vi "HighPassFilter.vi"(10 "Data":waveform(dbl)={"t0"=timestamp(3769531068.022168 s since 1904-01-01), "dt"=2.0833333333333333e-05, "Y"=array[14400 elements]}, 11 "Settings":T1={"Name of test"="Colin--Colin 01", "Date"=timestamp(3769531010.377861 s since 1904-01-01), "Location"="Home", "Template"="Acoustic Test", "Soundcard"="485B39 200083408035100798118210422", "resolution"=32, "Sampling rate"=48000, "Ch1 Gain "=0.0, "Ch2 Gain"=0.0, "Sample time (s)"=0.3, "Pre-trigger (s)"=0.001, "Hammer Threshold"=0.3, "Positions"=1, "Taps/Position"=5, "Set Names"="H", "Freq resolution"=1.0, "Hammer cutoff"=1.0, "Mic cutoff"=1.0, "Double bounce "=0.1, "Hammer Cal"=23.6, "dB Offset"=0.0, "Accel Cal"=1.0, "Vibrometer Cal"=40.0, "Mic Cal"=66.0, "Output"=2, "Voltage Cal"=1.0, "Vibrometer Port"="ASRL27::INSTR", "Range"=20, "High Pass"=2, "Bandwidth"=25, "X Range"=[{"Minimum"=200.0, "Maximum"=10000.0, "Increment"=10.0, "Minor Increment"=100.0, "Start"=200.0}, {"Minimum"=0.0005291005, "Maximum"=0.02, "Increment"=0.01, "Minor Increment"=0.001, "Start"=0.01}, {"Minimum"=0.0, "Maximum"=0.3, "Increment"=0.1, "Minor Increment"=0.01, "Start"=0.0}, {"Minimum"=200.0, "Maximum"=10000.0, "Increment"=10.0, "Minor Increment"=100.0, "Start"=1000.0}], "Y Range"=[{"Minimum"=-25.0, "Maximum"=0.0, "Increment"=5.0, "Minor Increment"=1.0, "Start"=-25.0}, {"Minimum"=-0.001, "Maximum"=0.01, "Increment"=0.002, "Minor Increment"=0.0005, "Start"=0.0}, {"Minimum"=-0.02, "Maximum"=0.02, "Increment"=0.01, "Minor Increment"=0.002, "Start"=-0.02}, {"Minimum"=-16.0, "Maximum"=24.0, "Increment"=2.0, "Minor Increment"=0.5, "Start"=-16.0}], "dB Spread"=40.0, "Trigger"=0, "Ch_1"=1, "Ch_2"=2, "flip?"=FALSE, "60Hz"=TRUE, "Time offset"=0.0, "Piezo Cal"=1.0, "Default Notes"=""} {"Ch_2" min=1 step=1; "Ch_1" min=1 max=100 step=1; "Trigger" items=["Hammer (force)", "Self-tap", "Spacebar"]; "Bandwidth" items=["1 kHz"=1, "5 kHz"=5, "10 kHz"=10, "25 kHz"=25, "50 kHz"=50, "100 kHz"=100]; "High Pass" items=["Off", "13 Hz", "104 Hz"]; "Range" items=["10 mm/s"=1, "20 mm/s"=2, "50 mm/s"=5, "100 mm/s"=10, "200 mm/s"=20, "500 mm/s"=50, "1 m/s"=100, "2 m/s"=200]; "Output" items=["Accelerometer", "Speed (from acceleration)", "Microphone", "Vibrometer", "Piezo"]; "Voltage Cal" format="%#_13g"; "Ch2 Gain" format="%#_13g"; "Ch1 Gain" format="%#_13g"; "Double bounce" min=0.0; "Mic cutoff" min=0.0 format="%#_4g"; "Hammer cutoff" min=0.0 format="%#_4g"; "Freq resolution" min=0.0; "Pre-trigger (s)" format="%#_13g"; "Date" format="%<%H:%M\n%d/%m/%y>T"; "resolution" items=["16 bit"=16, "24 bit"=24, "32 bit"=32]; "Sampling rate" items=["22050 samp/s"=22050, "44100 samp/s"=44100, "48000 samp/s"=48000]}) -> (1 "Data out":waveform(dbl)={"t0"=timestamp(3769531068.022168 s since 1904-01-01), "dt"=2.0833333333333333e-05, "Y"=array[14400 elements]}, 2 "Filtered X":dbl[](graph), 3 "dt":dbl=2.0833333333333333e-05)   [LabVIEW 2022 SP3]
uses:
  PreferencesControl.ctl
  <vilib>/Analysis/3filter.llb/Filter Passband Type.ctl
  <vilib>/Analysis/3filter.llb/Butterworth Filter (DBL).vi
  <vilib>/Analysis/NI_AALBase.lvlib
  <vilib>/Analysis/NI_AALPro.lvlib
  <vilib>/Analysis/2dsp.llb/Power Spectrum (DBL).vi
panel:
  out "Spectra":cluster{dbl, dbl, "Power Spectrum":dbl[]}[](graph)=[{0.0, 3.3333333333333335, "Power Spectrum"=array[14400 elements]}, {0.0, 3.3333333333333335, "Power Spectrum"=array[14400 elements]}]
  # "Hz"
  # "dB"
  # "dB"
  # "sec"
  # "sec"
  # "mV/Pa"
  # "mV/m/s2"
  # "mV/mm/s"
  # "V/N"
  # "sec"
  # "sec"
  # "mV/N"
  # "a.u."
  # "a.u."
  # "sec"
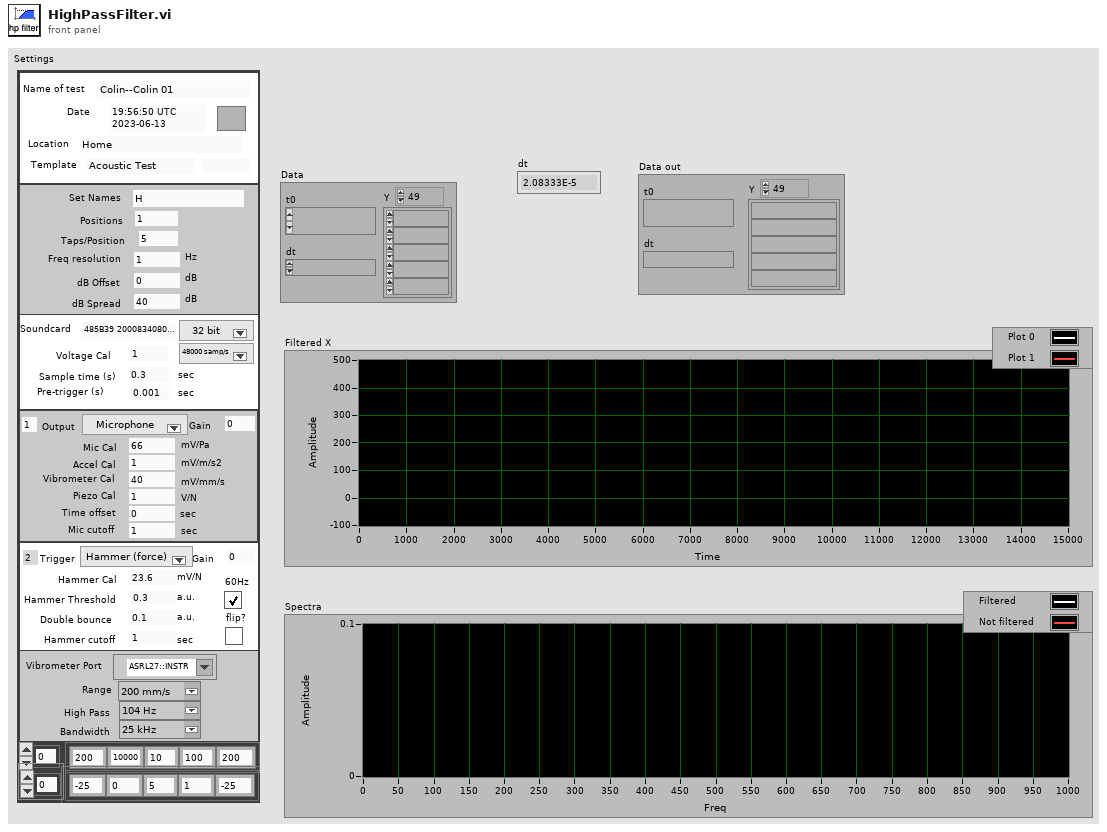
[diagram p1: front panel]
types:
  T1 = typedef "PreferencesControl.ctl" = cluster{"Name of test":string, "Date":timestamp, "Location":string, "Template":string, "Soundcard":string, "resolution":u16, "Sampling rate":u16, "Ch1 Gain ":dbl, "Ch2 Gain":dbl, "Sample time (s)":dbl, "Pre-trigger (s)":dbl, "Hammer Threshold":dbl, "Positions":i16, "Taps/Position":i16, "Set Names":string, "Freq resolution":dbl, "Hammer cutoff":dbl, "Mic cutoff":dbl, "Double bounce ":dbl, "Hammer Cal":dbl, "dB Offset":dbl, "Accel Cal":dbl, "Vibrometer Cal":dbl, "Mic Cal":dbl, "Output":u16, "Voltage Cal":dbl, "Vibrometer Port":refnum<visa-resource-name>, "Range":u16, "High Pass":u16, "Bandwidth":u16, "X Range":cluster{"Minimum":dbl, "Maximum":dbl, "Increment":dbl, "Minor Increment":dbl, "Start":dbl}[], "Y Range":cluster{"Minimum":dbl, "Maximum":dbl, "Increment":dbl, "Minor Increment":dbl, "Start":dbl}[], "dB Spread":dbl, "Trigger":u16, "Ch_1":u8, "Ch_2":u8, "flip?":bool, "60Hz":bool, "Time offset":dbl, "Piezo Cal":dbl, "Default Notes":string}
  T2 = typedef "NI_AALBase.lvlib/Filter Passband Type.ctl" = enum32{"Lowpass", "Highpass", "Bandpass", "Bandstop"}
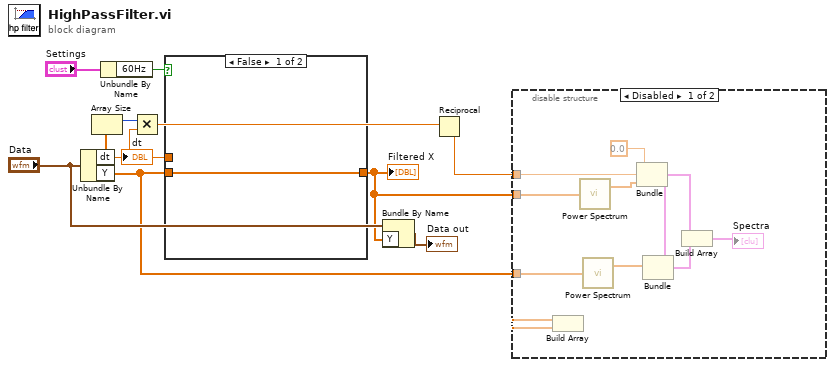
[diagram p0: block diagram]
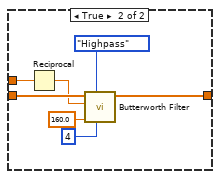
[diagram p3: hidden frame]
diagram:
  n1 = Unbundle By Name("Data") -> ("dt"=w7:dbl, "Y"=w2:dbl[])
  "dt" <- w7
  n2 = Array Size(array=w2) -> (size(s)=w8:i32)
  n3 = Unbundle By Name("Settings") -> ("60Hz"=w9:bool)
  n4 = Multiply(x=w8, y=w7) -> (x*y=w6:dbl)
  n5 = case shown="False" w9 {
    tunnel: w2 -> [w11 w18]
    tunnel: w7 -> [_ w17]
    tunnel: [w11 w12] -> w1
    frame False {
    }
    frame True {
      n6 = Reciprocal(x=w17) -> (1/x=w16:dbl)
      n7 = call-poly <vilib>:"Butterworth Filter.vi"("order"=4, "filter type"=Filter_Passband_Type."Highpass", "low cutoff freq: fl"=160.0, "sampling freq: fs"=w16, "X"=w18) -> ("Filtered X"=w12:dbl[])  [unwired: 3 in, 1 out]
    }
  }
  "Filtered X" <- w1
  n8 = Bundle By Name(cluster="Data", "Y"=w1) -> (→"Data out":waveform(dbl))
  n9 = Reciprocal(x=w6) -> (1/x=w5:dbl)
  n10 = disable-structure shown="Disabled" {
    disable-tunnel: w5 -> [w27 _]
    disable-tunnel: w2 -> [w20 _]
    disable-tunnel: w1 -> [w19 _]
    frame Disabled {
      n11 = Build Array(w20, w19) -> ()  [unwired: 1 out]
      n12 = call-poly <vilib>:"Power Spectrum.vi"("X"=w19) -> ("Power Spectrum"=w26:dbl[])  [unwired: 1 out]
      n13 = call-poly <vilib>:"Power Spectrum.vi"("X"=w20) -> ("Power Spectrum"=w25:dbl[])  [unwired: 1 out]
      n14 = Bundle(0.0, w27, "Power Spectrum"=w26) -> (w22:cluster{dbl, dbl, "Power Spectrum":dbl[]})  [unwired: 1 in]
      n15 = Bundle(cluster=w22, "Power Spectrum"=w25) -> (w21:cluster{dbl, dbl, "Power Spectrum":dbl[]})  [unwired: 2 in]
      n16 = Build Array(w22, w21) -> (→"Spectra":cluster{dbl, dbl, "Power Spectrum":dbl[]}[])
    }
    frame Enabled {
    }
  }
